vi "Acquisition.vi"(7 "Name(\"\" to use uuid)":string="Acquisition") -> ()   [LabVIEW 2017, in "Acquisition.lvlib"]
uses:
  Acquisition.lvlib
  _support/Hardware Configuration.ctl
  _support/Signal Type.ctl
  bc6f9ce3-7135-4df3-9fce-67397201bd09.vi
  f3e3012a-dc83-45d7-82c5-490bef76f43f.vi
  e2413101-be31-4c43-921b-7e7496268bc5.vi
  07cbb487-6694-43fd-ac53-f2be3466fcff.vi
  fecb174d-6823-407c-a974-ffebb4610b14.vi
  0bf643a1-791c-4b4c-b91f-da80b9c7e2fb.vi
  041ba748-83ae-40d3-86c4-8e2f4b565384.vi
  <userlib>/_NEVSTOP/Communicable State Machine(CSM)/AdvanceAPI/CSM - Revert Arguments-Safe String.vi
  <userlib>/_NEVSTOP/Communicable State Machine(CSM)/_Shared/Trim Single-line Text.vi
  <userlib>/_NEVSTOP/Communicable State Machine(CSM)/AdvanceAPI/CSM - Make String Arguments Safe.vi
  <userlib>/_NEVSTOP/Communicable State Machine(CSM)/AdvanceAPI/CSM - Break Down Multiple States String.vi
  <userlib>/_NEVSTOP/Communicable State Machine(CSM)/AdvanceAPI/CSM - Compact Multiple States.vi
  f3e3012a-dc83-45d7-82c5-490bef76f43f.vi/99de0c97-112a-4c86-9094-c187659127e1.vi
  <userlib>/_NEVSTOP/Communicable State Machine(CSM)/Utility/Build Error Cluster.vi
  0bf643a1-791c-4b4c-b91f-da80b9c7e2fb.vi/99de0c97-112a-4c86-9094-c187659127e1.vi
  <userlib>/_NEVSTOP/Communicable State Machine(CSM)/AdvanceAPI/CSM - Keywords.vi
  <vilib>/Utility/Data Type/Get Type Information.vi
  <userlib>/_NEVSTOP/Communicable State Machine(CSM)/addons/API-String-Arugments-Support/_Support/Data To SingleElementsArray_csm.vi
  <userlib>/_NEVSTOP/Communicable State Machine(CSM)/addons/API-String-Arugments-Support/_Support/Data To API String Arguments.vi
  <userlib>/_NEVSTOP/Communicable State Machine(CSM)/addons/INI-Static-Variable-Support/_Support/Parse Used Session and Name.vi
  <userlib>/_NEVSTOP/Communicable State Machine(CSM)/addons/INI-Static-Variable-Support/_Support/INI-FGV(lvlibp).vi
  <userlib>/_NEVSTOP/Communicable State Machine(CSM)/addons/INI-Static-Variable-Support/_Support/Populate String with INI Variable.vi
  <userlib>/_NEVSTOP/Communicable State Machine(CSM)/addons/API-String-Arugments-Support/_Support/Convert API String Arguments to Data(variant).vi
  <userlib>/_NEVSTOP/Communicable State Machine(CSM)/addons/API-String-Arugments-Support/_Support/SingleElementsArray To Data_csm.vi
  <userlib>/_NEVSTOP/Communicable State Machine(CSM)/addons/API-String-Arugments-Support/_Support/Query Data as API String Arguments(variant).vi
  <userlib>/_NEVSTOP/Communicable State Machine(CSM)/addons/MassData-Parameter/_support/FGV-MassData(lvlibp).vi
  <userlib>/_NEVSTOP/Communicable State Machine(CSM)/_Polymophic/Add State(s) to Queue By BOOL(Element).vi
  <userlib>/_NEVSTOP/Communicable State Machine(CSM)/_Polymophic/CSM - Filter Duplicated Lines.vi
  <userlib>/_NEVSTOP/Communicable State Machine(CSM)/_Polymophic/CSM - Replace Marks in Messages.vi
  <userlib>/_NEVSTOP/Communicable State Machine(CSM)/Communicable State Machine.lvlib
  <userlib>/_NEVSTOP/Communicable State Machine(CSM)/addons/Loop-Support/CSM Loop Support.lvlib
  <userlib>/_NEVSTOP/Communicable State Machine(CSM)/_Shared/CSM Shared.lvlib
panel:
  in  "Signal Type":enum16{"Sine Wave", "Square with Noise"}(ring)
  in  "Cancel Button":bool
  in  "OK Button":bool
  out "Error Occurred":errorcluster
  out "State History":string
  # "Configure The Simulated Waveform Type"
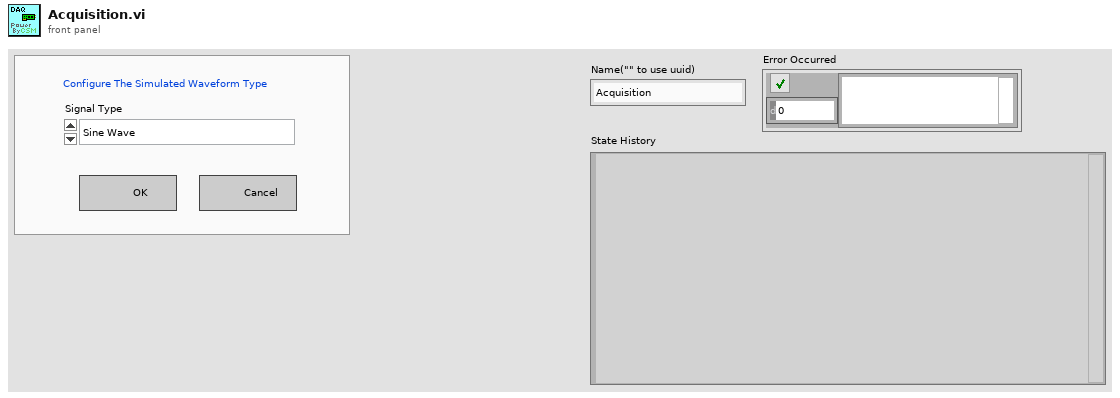
[diagram p1: front panel]
types:
  T1 = enum32{"Invalid", "Default", "Floating", "Floating/Auto-Hide", "Modal"}
  T2 = typedef "Acquisition.lvlib/Hardware Configuration.ctl" = cluster{"Resource":string, "SignalType":T3}
  T3 = typedef "Acquisition.lvlib/Signal Type.ctl" = enum16{"Sine Wave", "Square with Noise"}
  T4 = enum32{"Invalid", "Standard", "Closed", "Hidden", "Minimized", "Maximized"}
  T5 = enum32{"invalid app kind", "Development System", "Run Time System", "Student Edition", "Embedded LabVIEW", "Evaluation", "Custom"}
  T6 = typedef "Communicable State Machine.lvlib/_CSM_Response Source Message.ctl" = cluster{"‘State":string, "’Arguments":string, "’Error":errorcluster}
  T7 = cluster{"Current VI Reference":refnum<vi>, "Close Panel on Exit?":bool}
  T8 = cluster{"Core":cluster{"Current VI Reference":refnum<vi>, "Close Panel on Exit?":bool}, "Configuration":T2, "State":enum16{"Idle", "Acquiring"}, "SamplePeroid(ms)":u32}
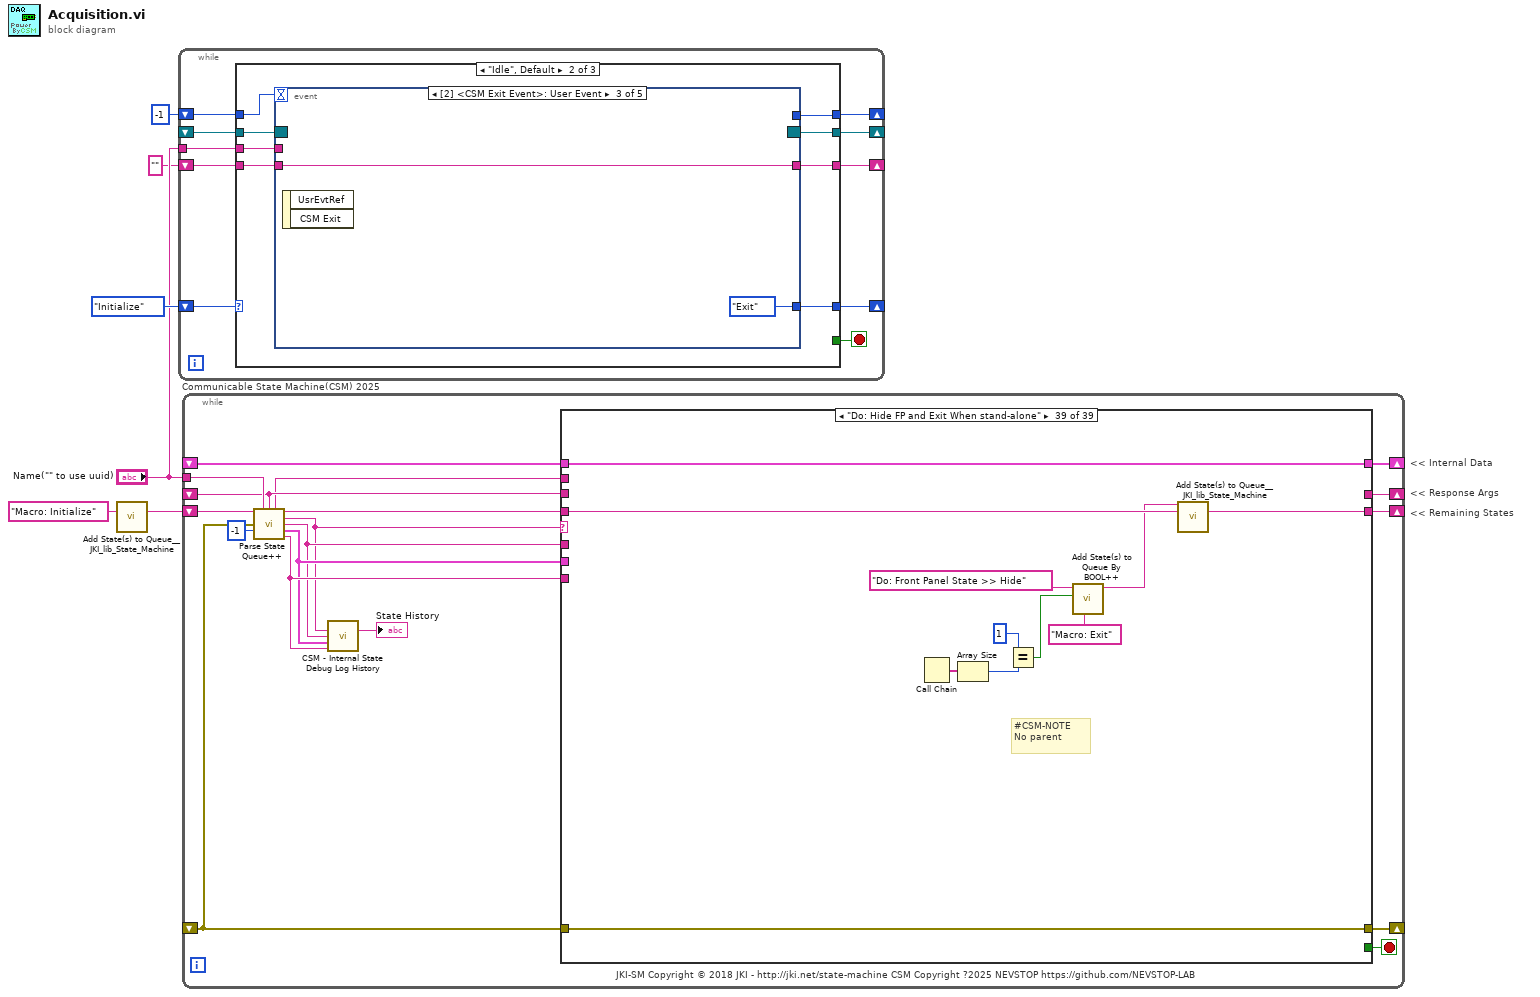
[diagram p0: block diagram]
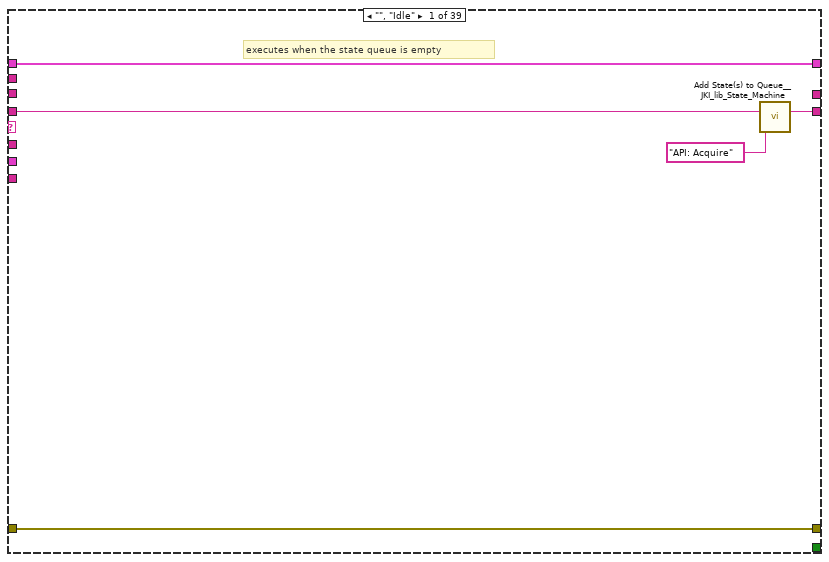
[diagram p2: hidden frame]
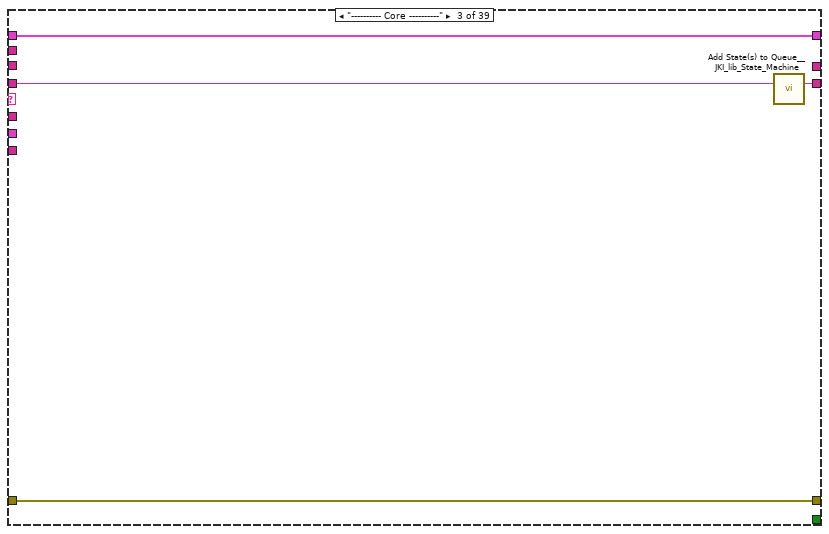
[diagram p4: hidden frame]
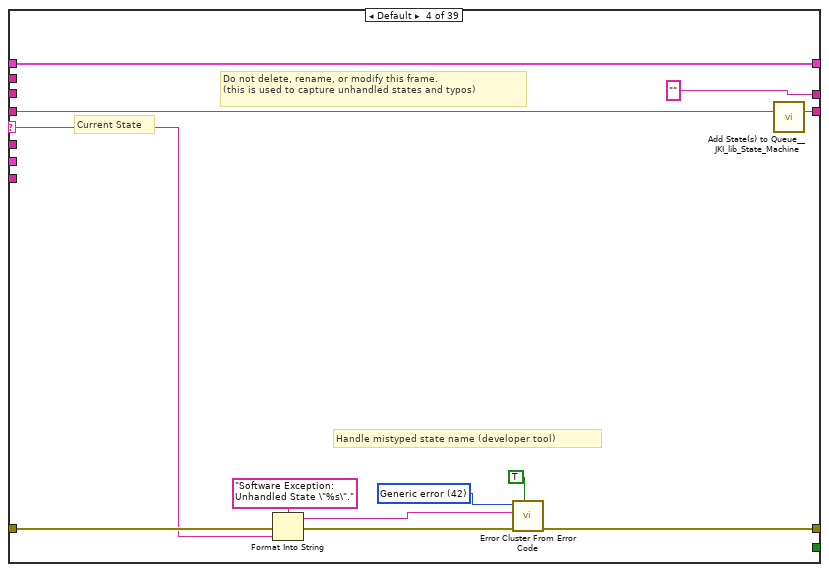
[diagram p5: hidden frame]
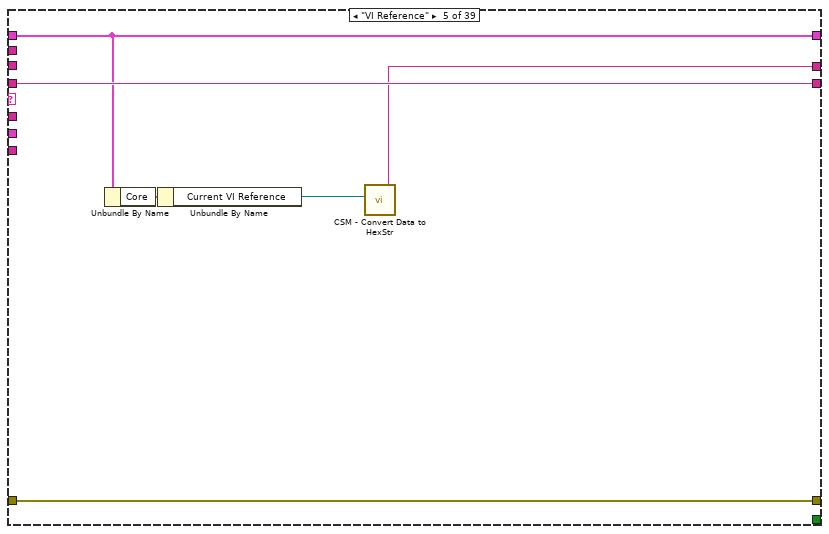
[diagram p6: hidden frame]
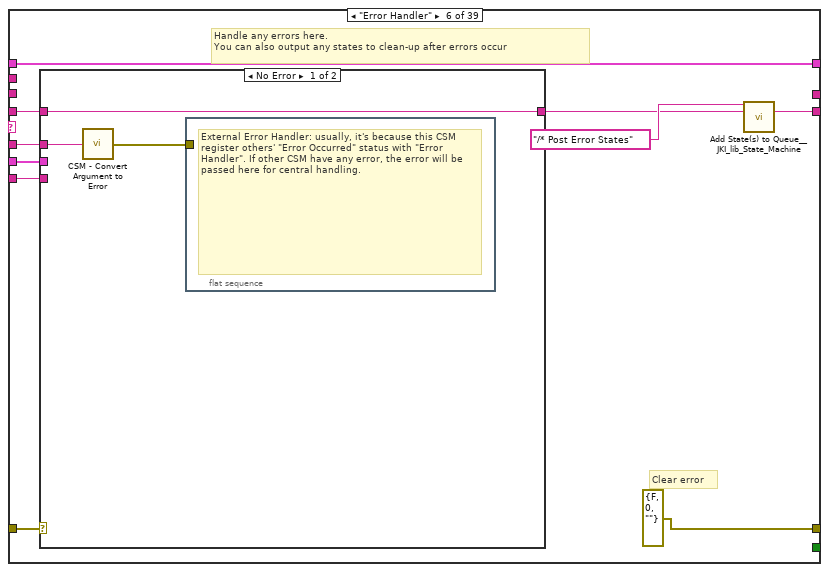
[diagram p7: hidden frame]
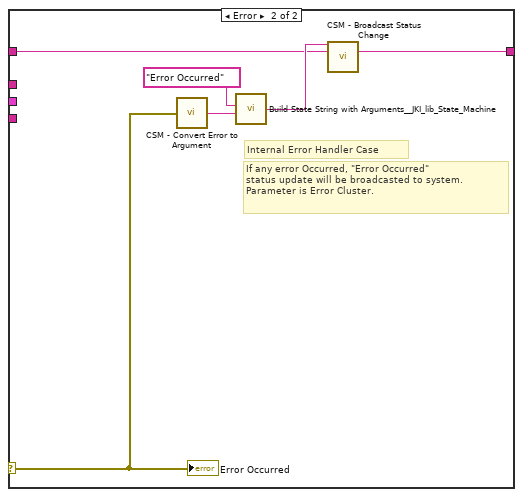
[diagram p8: hidden frame]
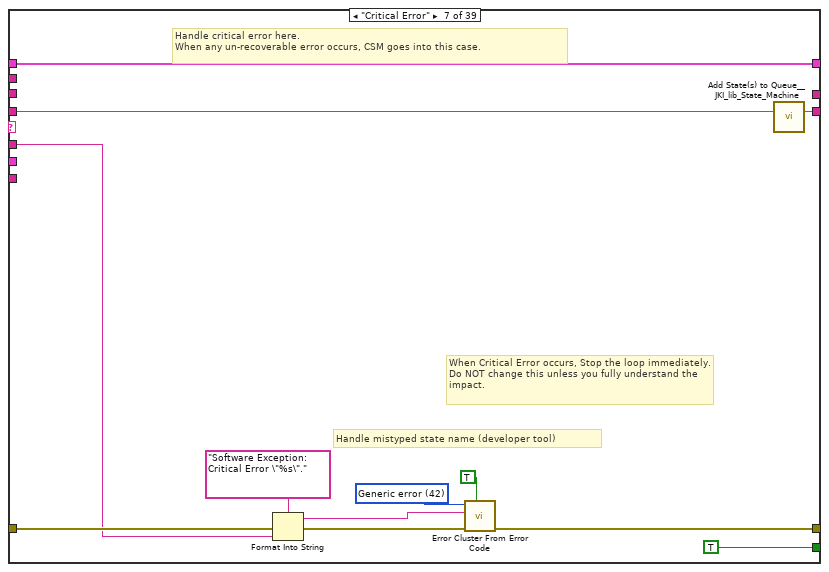
[diagram p9: hidden frame]
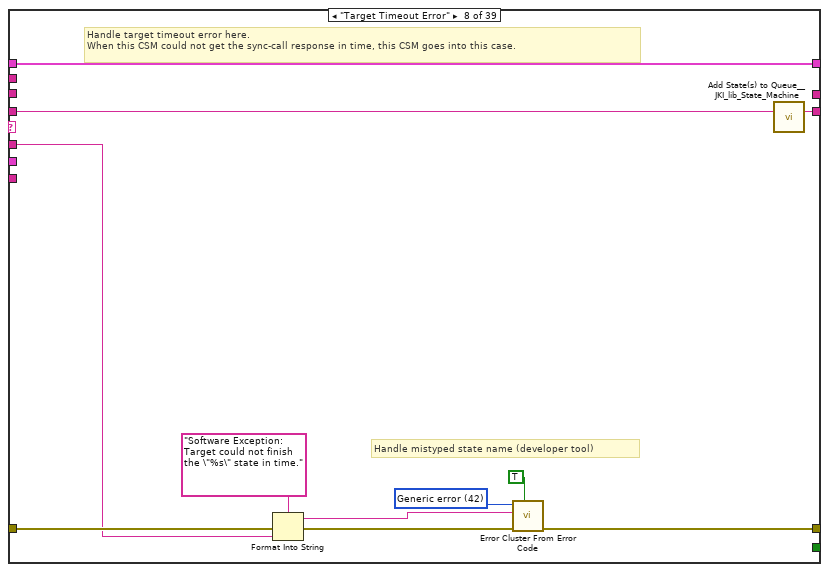
[diagram p10: hidden frame]
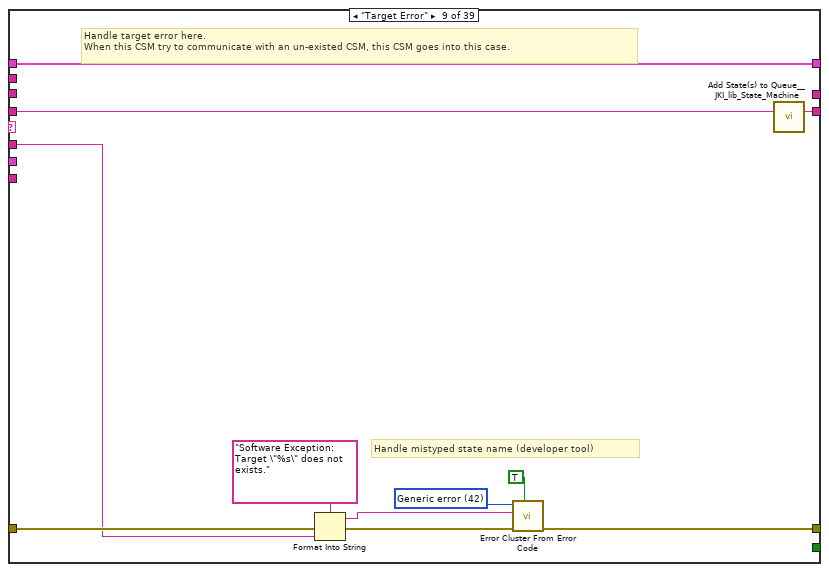
[diagram p11: hidden frame]
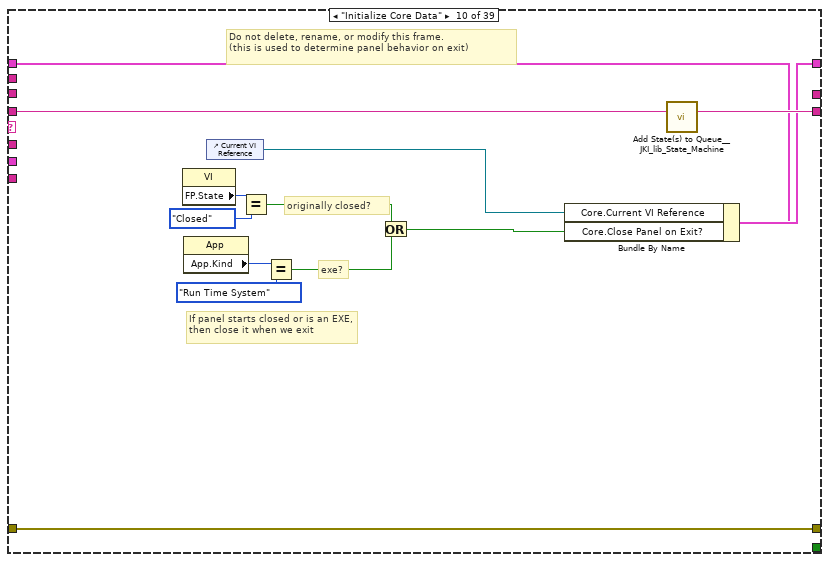
[diagram p12: hidden frame]
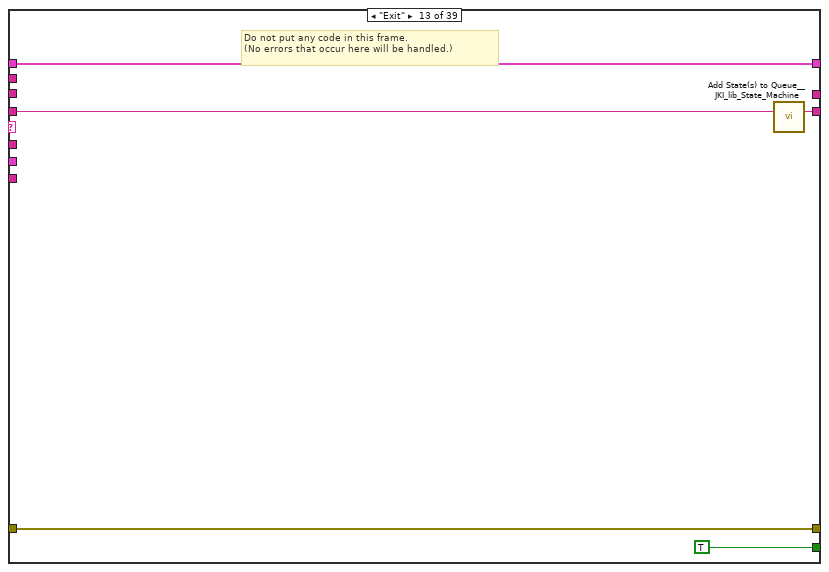
[diagram p15: hidden frame]
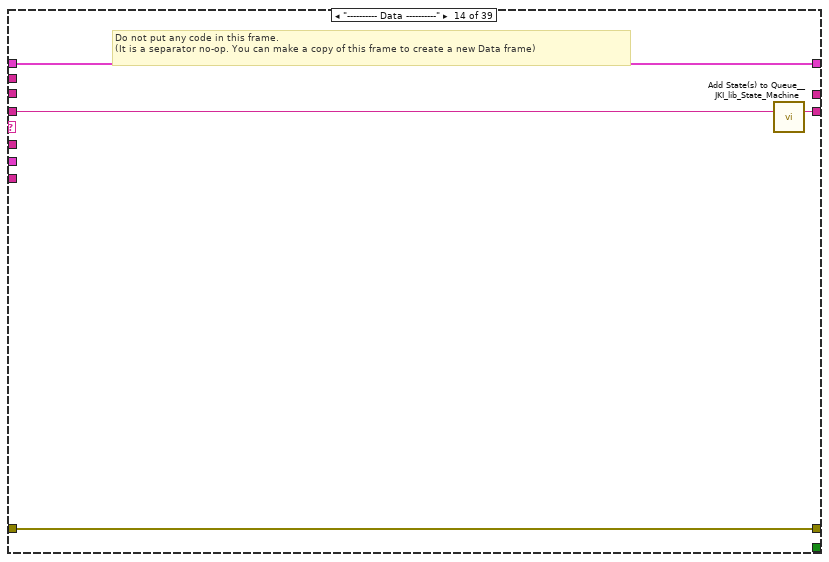
[diagram p16: hidden frame]
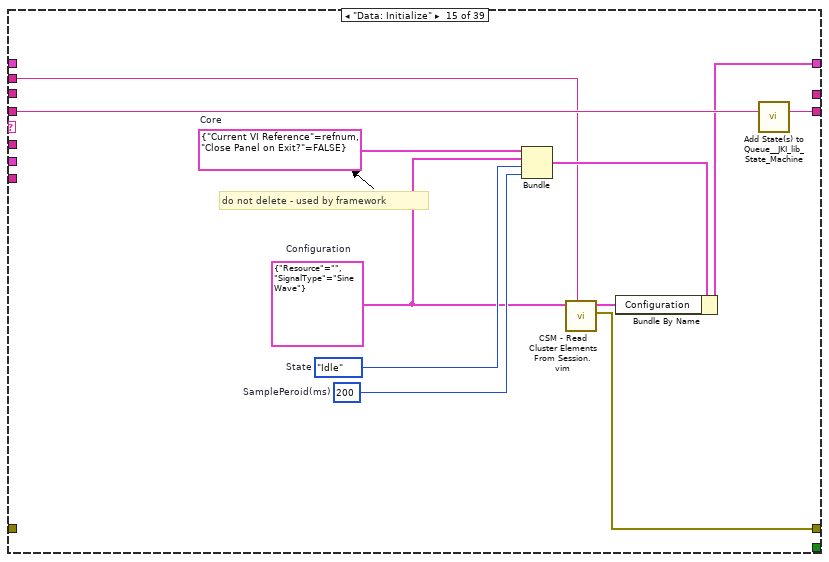
[diagram p17: hidden frame]
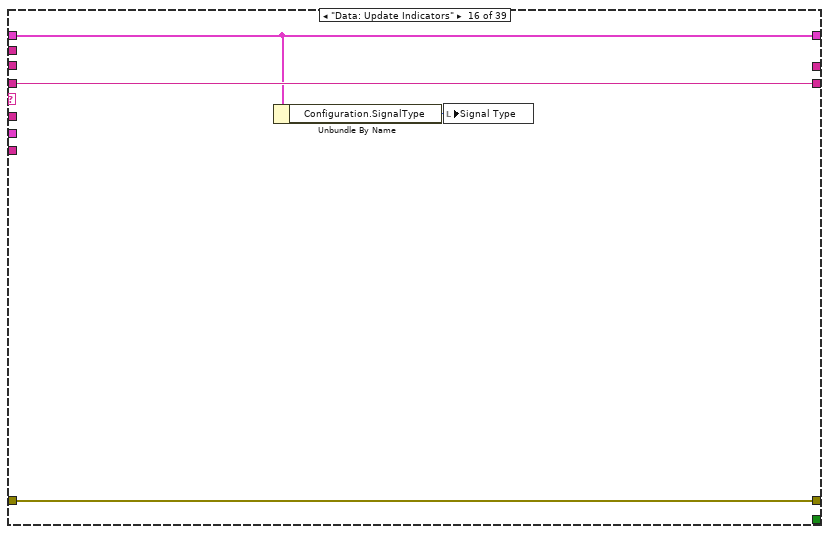
[diagram p18: hidden frame]
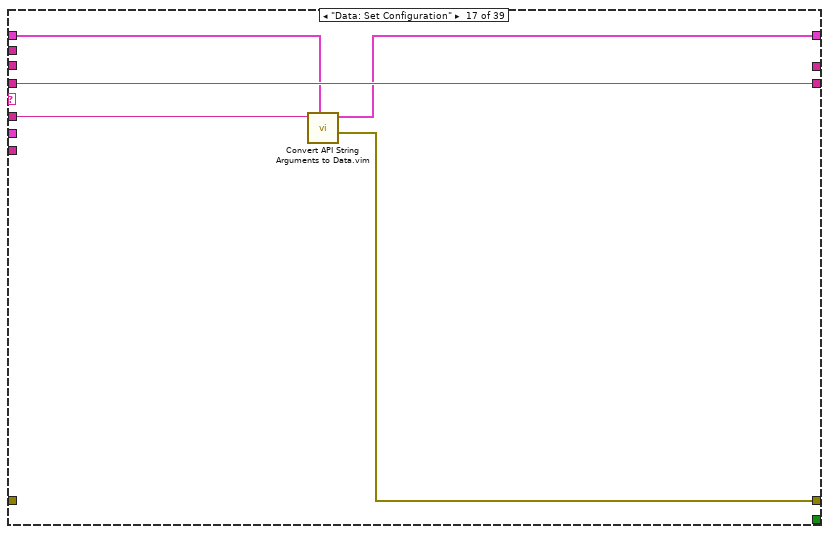
[diagram p19: hidden frame]
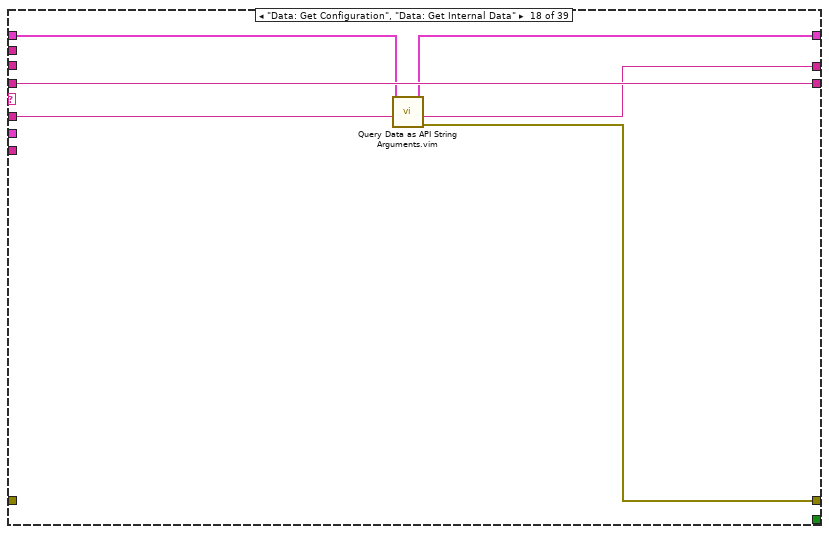
[diagram p20: hidden frame]
diagram:
  # "<< Internal Data"
  # "<< Response Args"
  # "<< Remaining States"
  n1 = call <vilib>:"Add State(s) to Queue__JKI_lib_State_Machine.vi"("State(s) in (\"\")"="Macro: Initialize") -> ("States Out"=w5:string)  [unwired: 14 in]
  n2 = while {
    shift-right: [w12] -> _
    shift-left: enum16{"Idle", "Initialize", "Exit"}."Initialize" -> [w16]
    tunnel: "Name(\"\" to use uuid)" -> [w15]
    shift-right: [w14] -> _
    shift-left: _ -> [w13]
    shift-right: [w9] -> _
    shift-left: "" -> [w10]
    shift-right: [w7] -> _
    shift-left: -1 -> [w8]
    stop <- w11 stop-if-true
    n3 = case shown="\"Idle\", Default" w16 {
      tunnel: w15 -> [w25 w29 _]
      tunnel: [w22 w34 _] -> w14
      tunnel: w13 -> [_ w33 w62]
      tunnel: [enum16{"Idle", "Initialize", "Exit"}."Idle" w32 _] -> w12
      tunnel: [_ _ TRUE] -> w11
      tunnel: w10 -> [w19 w31 w59]
      tunnel: [w19 w30 w59] -> w9
      tunnel: w8 -> [w18 w27 w58]
      tunnel: [w18 w28 w58] -> w7
      frame "Initialize" {
        n4 = call <userlib>:"CSM - Wait for Module to Be Alive.vi"("CSM Name"=w25) -> ("CSM Name (Dup)"=w20:string, "error out"=w26:errorcluster)  [unwired: 12 in, 1 out]
        n5 = call <userlib>:"CSM - Module Exit Event.vi"("Error In"=w26, "Name (\"\" to Use UUID) In"=w20) -> ("error out"=w24:errorcluster, "CSM Exit Event"=w23:refnum<user-event>)  [unwired: 7 in, 1 out]
        n6 = register-events(error in=w24, w23) -> (reference out=w22:refnum<event-registration>)  [unwired: 1 in, 1 out]
        n7 = property class="VI"("FP.Behavior"=T1."Default" ("Front Panel Window:Behavior")) -> ()  [unwired: 2 in, 2 out]
      }
      frame "Idle", Default {
        n8 = event shown="[2] <CSM Exit Event>: User Event" {
          selector: w33 -> [_ _ _ _ _]
          dyn-events: [_ _ _ _ _] -> w34
          timeout: w27 -> [_ _ _ _ _]
          tunnel: [_ _ enum16{"Idle", "Initialize", "Exit"}."Exit" _ _] -> w32
          tunnel: w31 -> [w38 w42 w44 w53 w56]
          tunnel: [w39 w41 w44 w52 w55] -> w30
          tunnel: w29 -> [w36 _ _ _ _]
          tunnel: [-1 _ _ _ _] -> w28
          event Timeout {
            n9 = event-data() -> ()  [unwired: 1 in, 3 out]
            n10 = call-poly <userlib>:"CSM - Filter JKISM String Queue.vi"("States In"=w38) -> ("States Out"=w35:string)  [unwired: 14 in]
            n11 = call <userlib>:"CSM - Forward UI Operations to CSM.vi"("Name (\"\" to Use UUID)"=w36, "State(s) In (\"\")"=w35) -> ("States Out"=w39:string)  [unwired: 8 in, 1 out]
          }
          event Panel Close? {
            n12 = event-data() -> ()  [unwired: 1 in, 2 out]
            n13 = call <vilib>:"Add State(s) to Queue__JKI_lib_State_Machine.vi"("State(s) in Front (\"\")"="Do: Hide FP and Exit When stand-alone" ("State(s) in Front (\"\")"), "State(s) in (\"\")"=w42) -> ("States Out"=w41:string)  [unwired: 13 in]
            n14 = event-data("Discard?"=TRUE) -> ()  [unwired: 1 in, 1 out]
          }
          event User Event {
            n15 = event-data() -> ()  [unwired: 1 in, 2 out]
          }
          event "OK Button": Value Change {
            n16 = event-data() -> ()  [unwired: 1 in, 1 out]
            n17 = Bundle By Name(cluster=T2 {"Resource"="", "SignalType"=enum."Sine Wave"} ("Hardware Config"), "SignalType"="Signal Type") -> (w48:T2)
            n18 = call "Convert Data To API String Arguments.vim"("Data"=w48) -> ("API String"=w47:string)  [unwired: 7 in, 1 out]
            n19 = call-poly <userlib>:"Build Message with Arguments++.vi"("States With Replace Token"="API: Update Settings >> <param>\nData: Update Indicators\nDo: Hide FP and Exit When stand-alone" ("State"), "<param>"=w47) -> ("States"=w46:string)  [unwired: 13 in]
            n20 = call <vilib>:"Add State(s) to Queue__JKI_lib_State_Machine.vi"("State(s) in (\"\")"=w53, "State(s) at Back (\"\")"=w46) -> ("States Out"=w52:string)  [unwired: 13 in]
          }
          event "Cancel Button": Value Change {
            n21 = event-data() -> ()  [unwired: 1 in, 1 out]
            n22 = call <vilib>:"Add State(s) to Queue__JKI_lib_State_Machine.vi"("State(s) in Front (\"\")"="Do: Hide FP and Exit When stand-alone" ("State(s) in Front (\"\")"), "State(s) in (\"\")"=w56) -> ("States Out"=w55:string)  [unwired: 13 in]
          }
        }
      }
      frame "Exit" {
        n23 = Unregister For Events(event registration refnum=w62) -> (error out=w61:errorcluster)  [unwired: 1 in]
        n24 = call <vilib>:"Clear Errors.vi"("error in (no error)"=w61) -> ()  [unwired: 5 in, 2 out]
        n25 = property class="VI"("FP.Behavior"=T1."Default" ("Front Panel Window:Behavior")) -> ()  [unwired: 2 in, 2 out]
      }
    }
  }
  n26 = while "Communicable State Machine(CSM) 2025" {
    shift-right: [w75] -> _
    shift-left: _ -> [w65]
    shift-right: [w78] -> _
    shift-left: _ -> [w74]
    shift-right: [w77] -> _
    shift-left: w5 -> [w79]
    tunnel: "Name(\"\" to use uuid)" -> [w72]
    shift-right: [w73] -> _
    shift-left: _ -> [w67]
    stop <- w76 stop-if-true
    # "JKI-SM Copyright © 2018 JKI - http://jki.net/state-machine CSM Copyright ?2025 NEVSTOP https://github.com/NEVSTOP-LAB"
    n27 = call <userlib>:"Parse State Queue++.vi"("State Queue"=w79, "Name (\"\" to Use UUID)"=w72, "Response Arguments"=w67, "Previous Error"=w74, "Dequeue (1 ms)"=-1 ("Dequeue Timeout(1ms)")) -> ("Name Used"=w66:string, "Remaining States"=w80:string, "Current State"=w68:string, "Arguments"=w69:string, "Additional Information"=w70:T6, "Source CSM"=w71:string)  [unwired: 5 in]
    n28 = call <userlib>:"CSM - Internal State Debug Log History.vi"("State"=w68, "Arguments (\"\")"=w69, ">> Response Source Message >>"=w70, "Source (\"\")"=w71) -> ("Debug Log"=→"State History":string)  [unwired: 11 in]
    n29 = case shown="\"Do: Hide FP and Exit When stand-alone\"" w68 {
      selector: w68 -> [_ _ _ w94 _ _ _ _ _ _ _ _ _ _ _ _ _ _ _ _ _ _ _ _ _ _ _ _ _ _ _ _ _ _ w334 _ _ _ _]
      tunnel: w80 -> [w82 w87 w92 w98 w109 w114 w135 w147 w158 w176 w178 w181 w187 w191 w202 w205 w211 w217 w223 w227 w232 w237 w239 w243 w256 w269 w280 w287 w293 w298 w303 w326 w328 w331 w338 w341 w345 w352 w419]
      tunnel: w69 -> [_ _ _ _ _ w113 w131 w143 w154 _ _ _ _ _ _ _ w209 w214 _ _ _ _ _ _ _ w265 _ _ _ _ _ _ _ _ w333 _ _ w349 _]
      tunnel: w65 -> [w84 w86 w89 w96 w108 w119 w133 w145 w156 w169 w177 w180 w185 w188 _ w203 w210 w216 w218 w224 w229 w234 w238 w246 w252 w267 w279 w285 w290 w297 w305 w323 w327 w330 w336 w342 w344 w351 w428]
      tunnel: [w85 w88 w90 w100 w110 errorcluster {"status"=FALSE, "code"=0, "source"=""} ("error out") w137 w142 w153 w173 w179 w182 w184 w189 w192 w206 w207 w212 w219 w225 w230 w235 w240 w244 w254 w261 w281 w282 w288 w299 w307 w324 w329 w332 w339 w343 w346 w348 w427] -> w78
      tunnel: w74 -> [w85 w88 w90 w99 w110 w117 w136 w148 w159 w173 w179 w182 w184 w189 _ w206 _ _ w220 w225 w230 w235 w240 w244 w254 _ w281 _ _ w299 w308 _ w329 w332 w339 w343 w346 w350 w427]
      tunnel: [w83 w87 w91 w97 w109 w115 w134 w146 w157 w175 w178 w181 w186 w190 w201 w205 w211 w217 w222 w226 w231 w236 w239 w242 w255 w269 w280 w287 w293 w298 w304 w326 w328 w331 w337 w340 w345 w352 w420] -> w77
      tunnel: [_ _ _ _ _ _ TRUE _ _ _ _ _ TRUE _ _ _ _ _ _ _ _ _ _ _ _ _ _ _ _ _ _ _ _ _ _ _ _ _ _] -> w76
      tunnel: [w84 w86 w89 w96 w108 w119 w133 w145 w156 w174 w177 w180 w185 w188 w194 w203 w208 w215 w218 w224 w229 w234 w238 w245 w252 w268 w279 w283 w289 w296 w306 w322 w327 w330 w336 w342 w344 w351 w428] -> w75
      tunnel: w71 -> [_ _ _ _ _ w112 _ _ _ _ _ _ _ _ _ _ _ _ _ _ _ _ _ _ _ _ _ _ _ _ _ _ _ _ _ _ _ _ _]
      tunnel: w70 -> [_ _ _ _ _ w111 _ _ _ _ _ _ _ _ _ _ _ _ _ _ _ _ _ _ _ _ _ _ _ _ _ _ _ _ _ _ _ _ _]
      tunnel: [_ _ _ "" w105 _ _ _ _ _ _ _ _ _ _ _ _ w213 _ _ _ _ _ _ _ _ _ _ _ _ w301 _ _ _ _ _ _ _ _] -> w73
      tunnel: w66 -> [_ _ _ _ _ _ _ _ _ _ _ _ _ _ w196 _ _ _ _ _ _ _ _ _ _ w260 _ _ _ _ _ _ _ _ _ _ _ _ _]
      tunnel: w67 -> [_ _ _ _ _ _ _ _ _ _ _ _ _ _ _ _ _ _ _ _ _ _ _ _ _ _ _ _ _ _ _ _ _ _ _ _ _ _ _]
      frame "", "Idle" {
        # "executes when the state queue is empty"
        n30 = call <vilib>:"Add State(s) to Queue__JKI_lib_State_Machine.vi"("State(s) in (\"\")"=w82, "State(s) at Back (\"\")"="API: Acquire" ("State(s) in Front (\"\")")) -> ("States Out"=w83:string)  [unwired: 13 in]
      }
      frame "CSM Documentation" {
        # "CSM Documentation"
        # "State Syntax:\nStateCategory: State >> Argument -@ CSMName\nStateCategory: State >> Argument -> CSMName\n\nLine Terminator: Line feed"
        # "Commenting:\nTo add a comment use \"//\" or \"#\" and all text to the right will be ignored\nCommenting Example:\nUI: Initialize // This initializes the UI\n// Another comment line"
        # "Example:\nUI: Help >> About -@Main\nUI: Help >> About ->Main\n\nWhere \"UI\" is the state category\nWhere \"Help\" is the state\nWhere \"About\" is the argument\nWhere \"Main\" is the Name of CSM,which actually run the \"UI: Help >> About\"\n\n    \"-@\" stands for sync state. Current CSM will wait until the state is finished. \n            - if \"Main\" named CSM does not exist, \"Target Error\" will occur.\n            - if \"Main\" named CSM is in another sync remote state, \"Target Busy Error\" will occur.\n            - if \"Main\" named CSM could not finish the state in time, \"Target Timeout Error\" will occur.\n            - if everything is right. \"Response\" will occur with Argument back from \"Main\" named CSM. \n\n    \"->\" stands for async state. Current CSM will post the state and continue to next state in next iteration.\n            - if \"Main\" named CSM does not exist, \"Target Error\" will occur.\n            - if everything is right. \"Async Message Posted\" will occur.\n            - After State is finished. Caller will receive a \"Async Response\" state from callee.\n\nWhen duplicated name is used for multiple CSM module or some framework problem happens, \"Critical Error\" will occur."
      }
      frame "---------- Core ----------" {
        n31 = call <vilib>:"Add State(s) to Queue__JKI_lib_State_Machine.vi"("State(s) in (\"\")"=w92) -> ("States Out"=w91:string)  [unwired: 14 in]
      }
      frame Default {
        w103 = 42 items=["No error", "Argument error", "Memory is full", "Out of zone", "End of file", "File already open", "Generic file I/O error", "File not found", "File permission error", "Disk is full", "Duplicate path", "Too many files open", "System feature not enabled", "Resource file not found", "Cannot add resource", "Resource not found", "Image not found", "Image memory error", "Pen does not exist", "Config type invalid", "Config token not found", "Config parse error", "Config memory error", "Bad external code format", "Bad external code offset", "External code not present", "Null window", "Destroy window error", "Null menu", "Print aborted", "Bad print record", "Print driver error", "Windows error during printing", "Memory error during printing", "Print dialog error", "Generic print error", "Invalid device refnum", "Device not found", "Device parameter error", "Device unit error", "Cannot open device", "Device call aborted", "Generic error", "Cancelled by user", "Object ID too low", "Object ID too high", "Object not in heap", "Unknown heap", "Unknown object (invalid DefProc)", "Unknown object (DefProc not in table)", "Message out of range", "Invalid (null) method", "Unknown message", "Manager call not supported", "Bad address", "Network operation in progress", "Network operation timed out", "Connection is busy", "Network attribute not supported", "Network error", "Address in use", "System out of memory", "Connection aborted", "Connection refused", "Not connected", "Already connected", "Connection closed", "Initialization error (interapplication manager)", "Bad occurrence", "Wait on unbound occurrence handler", "Occurrence queue overflow", "Datalog type conflict", "Unused", "Unrecognized type (interapplication manager)", "Memory corrupt", "Failed to make temporary DLL", "Old CIN version", "Drag socket not found", "Failed to load drop-object", "Failed to register OLE object", "Failed to release OLE object", "Format specifier type mismatch", "Unknown format specifier", "Too few format specifiers", "Too many format specifiers", "Scan failed", "Newer CIN version", "Error converting to variant", "Runtime menu error", "Password tampered", "Variant attribute not found", "Incompatible variant data type", "Event data is not available", "Event Store is not present", "Occurrence is not found", "Event Queue is not created", "Event info is not available", "Refnum passed is NULL", "Error retrieving Class GUID", "Error retrieving CoClass GUID", "Error retrieving TypeLib GUID.", "Bad built application magic bytes.", "Specific driver is different from the specific driver associated with the Logical Name.", "There is no session opened to the class driver.", "Max Error", "MAX - Error with config objects", "MAX - Error loading configuration", "MAX - Group not supported"]
        # "Current State"
        # "Do not delete, rename, or modify this frame.\n(this is used to capture unhandled states and typos)"
        # "Handle mistyped state name (developer tool)"
        n32 = Format Into String(format string="Software Exception: Unhandled State \"%s\"." ("message"), error in=w99, w94) -> (resulting string=w102:string, error out=w101:errorcluster)  [unwired: 1 in]
        n33 = call <vilib>:"Error Cluster From Error Code.vi"("show call chain? (False)"=TRUE, "error in (no error)"=w101, "error message (\"\")"=w102, "error code (0)"=w103) -> ("error out"=w100:errorcluster)  [unwired: 5 in]
        n34 = call <vilib>:"Add State(s) to Queue__JKI_lib_State_Machine.vi"("State(s) in (\"\")"=w98) -> ("States Out"=w97:string)  [unwired: 14 in]
      }
      frame "VI Reference" {
        n35 = Unbundle By Name(w108) -> ("Core"=w107:T7)
        n36 = Unbundle By Name(w107) -> ("Current VI Reference"=w106:refnum<vi>)
        n37 = call <userlib>:"CSM - Convert Data to HexStr.vi"("Variant"=w106) -> ("HEX String (0-9,A-F)"=w105:string)  [unwired: 8 in]
      }
      frame "Error Handler" {
        # "Handle any errors here.\nYou can also output any states to clean-up after errors occur"
        # "Clear error"
        n38 = case shown="No Error" w117 {
          selector: w117 -> [_ w124]
          tunnel: [w123 w126] -> w116
          tunnel: w114 -> [w123 w125]
          tunnel: w113 -> [w122 _]
          tunnel: w112 -> [_ _]
          tunnel: w111 -> [_ _]
          frame No Error {
            n39 = call <userlib>:"CSM - Convert Argument to Error.vi"("Argument"=w122) -> ("Error"=w121:errorcluster)  [unwired: 4 in]
            n40 = flat-sequence {
              tunnel: w121 -> [_]
              frame #0 {
                # "External Error Handler: usually, it's because this CSM register others' \"Error Occurred\" status with \"Error Handler\". If other CSM have any error, the error will be passed here for central handling."
              }
            }
          }
          frame Error {
            # "Internal Error Handler Case"
            # "If any error Occurred, \"Error Occurred\" \nstatus update will be broadcasted to system.\nParameter is Error Cluster."
            n41 = call <userlib>:"CSM - Convert Error to Argument.vi"("Error"=w124) -> ("Argument"=w128:string)  [unwired: 4 in]
            n42 = call <vilib>:"Build State String with Arguments__JKI_lib_State_Machine.vi"("Arguments (\"\")"=w128, "State"="Error Occurred" ("Status with Arguments")) -> ("State with Arguments"=w127:string)  [unwired: 4 in]
            n43 = call <userlib>:"CSM - Broadcast Status Change.vi"("Status With Arguments"=w127, "State Queue"=w125) -> ("Remaining States"=w126:string)  [unwired: 13 in]
            "Error Occurred" <- w124
          }
        }
        n44 = call <vilib>:"Add State(s) to Queue__JKI_lib_State_Machine.vi"("State(s) in Front (\"\")"="/* Post Error States", "State(s) in (\"\")"=w116) -> ("States Out"=w115:string)  [unwired: 13 in]
      }
      frame "Critical Error" {
        w140 = 42 items=["No error", "Argument error", "Memory is full", "Out of zone", "End of file", "File already open", "Generic file I/O error", "File not found", "File permission error", "Disk is full", "Duplicate path", "Too many files open", "System feature not enabled", "Resource file not found", "Cannot add resource", "Resource not found", "Image not found", "Image memory error", "Pen does not exist", "Config type invalid", "Config token not found", "Config parse error", "Config memory error", "Bad external code format", "Bad external code offset", "External code not present", "Null window", "Destroy window error", "Null menu", "Print aborted", "Bad print record", "Print driver error", "Windows error during printing", "Memory error during printing", "Print dialog error", "Generic print error", "Invalid device refnum", "Device not found", "Device parameter error", "Device unit error", "Cannot open device", "Device call aborted", "Generic error", "Cancelled by user", "Object ID too low", "Object ID too high", "Object not in heap", "Unknown heap", "Unknown object (invalid DefProc)", "Unknown object (DefProc not in table)", "Message out of range", "Invalid (null) method", "Unknown message", "Manager call not supported", "Bad address", "Network operation in progress", "Network operation timed out", "Connection is busy", "Network attribute not supported", "Network error", "Address in use", "System out of memory", "Connection aborted", "Connection refused", "Not connected", "Already connected", "Connection closed", "Initialization error (interapplication manager)", "Bad occurrence", "Wait on unbound occurrence handler", "Occurrence queue overflow", "Datalog type conflict", "Unused", "Unrecognized type (interapplication manager)", "Memory corrupt", "Failed to make temporary DLL", "Old CIN version", "Drag socket not found", "Failed to load drop-object", "Failed to register OLE object", "Failed to release OLE object", "Format specifier type mismatch", "Unknown format specifier", "Too few format specifiers", "Too many format specifiers", "Scan failed", "Newer CIN version", "Error converting to variant", "Runtime menu error", "Password tampered", "Variant attribute not found", "Incompatible variant data type", "Event data is not available", "Event Store is not present", "Occurrence is not found", "Event Queue is not created", "Event info is not available", "Refnum passed is NULL", "Error retrieving Class GUID", "Error retrieving CoClass GUID", "Error retrieving TypeLib GUID.", "Bad built application magic bytes.", "Specific driver is different from the specific driver associated with the Logical Name.", "There is no session opened to the class driver.", "Max Error", "MAX - Error with config objects", "MAX - Error loading configuration", "MAX - Group not supported"]
        # "Handle critical error here.\nWhen any un-recoverable error occurs, CSM goes into this case."
        # "When Critical Error occurs, Stop the loop immediately. Do NOT change this unless you fully understand the impact."
        # "Handle mistyped state name (developer tool)"
        n45 = Format Into String(format string="Software Exception: Critical Error \"%s\"." ("message"), error in=w136, w131) -> (resulting string=w139:string, error out=w138:errorcluster)  [unwired: 1 in]
        n46 = call <vilib>:"Error Cluster From Error Code.vi"("show call chain? (False)"=TRUE, "error in (no error)"=w138, "error message (\"\")"=w139, "error code (0)"=w140) -> ("error out"=w137:errorcluster)  [unwired: 5 in]
        n47 = call <vilib>:"Add State(s) to Queue__JKI_lib_State_Machine.vi"("State(s) in (\"\")"=w135) -> ("States Out"=w134:string)  [unwired: 14 in]
      }
      frame "Target Timeout Error" {
        w151 = 42 items=["No error", "Argument error", "Memory is full", "Out of zone", "End of file", "File already open", "Generic file I/O error", "File not found", "File permission error", "Disk is full", "Duplicate path", "Too many files open", "System feature not enabled", "Resource file not found", "Cannot add resource", "Resource not found", "Image not found", "Image memory error", "Pen does not exist", "Config type invalid", "Config token not found", "Config parse error", "Config memory error", "Bad external code format", "Bad external code offset", "External code not present", "Null window", "Destroy window error", "Null menu", "Print aborted", "Bad print record", "Print driver error", "Windows error during printing", "Memory error during printing", "Print dialog error", "Generic print error", "Invalid device refnum", "Device not found", "Device parameter error", "Device unit error", "Cannot open device", "Device call aborted", "Generic error", "Cancelled by user", "Object ID too low", "Object ID too high", "Object not in heap", "Unknown heap", "Unknown object (invalid DefProc)", "Unknown object (DefProc not in table)", "Message out of range", "Invalid (null) method", "Unknown message", "Manager call not supported", "Bad address", "Network operation in progress", "Network operation timed out", "Connection is busy", "Network attribute not supported", "Network error", "Address in use", "System out of memory", "Connection aborted", "Connection refused", "Not connected", "Already connected", "Connection closed", "Initialization error (interapplication manager)", "Bad occurrence", "Wait on unbound occurrence handler", "Occurrence queue overflow", "Datalog type conflict", "Unused", "Unrecognized type (interapplication manager)", "Memory corrupt", "Failed to make temporary DLL", "Old CIN version", "Drag socket not found", "Failed to load drop-object", "Failed to register OLE object", "Failed to release OLE object", "Format specifier type mismatch", "Unknown format specifier", "Too few format specifiers", "Too many format specifiers", "Scan failed", "Newer CIN version", "Error converting to variant", "Runtime menu error", "Password tampered", "Variant attribute not found", "Incompatible variant data type", "Event data is not available", "Event Store is not present", "Occurrence is not found", "Event Queue is not created", "Event info is not available", "Refnum passed is NULL", "Error retrieving Class GUID", "Error retrieving CoClass GUID", "Error retrieving TypeLib GUID.", "Bad built application magic bytes.", "Specific driver is different from the specific driver associated with the Logical Name.", "There is no session opened to the class driver.", "Max Error", "MAX - Error with config objects", "MAX - Error loading configuration", "MAX - Group not supported"]
        # "Handle target timeout error here.\nWhen this CSM could not get the sync-call response in time, this CSM goes into this case."
        # "Handle mistyped state name (developer tool)"
        n48 = Format Into String(format string="Software Exception: Target could not finish the \"%s\" state in time." ("message"), error in=w148, w143) -> (resulting string=w150:string, error out=w149:errorcluster)  [unwired: 1 in]
        n49 = call <vilib>:"Error Cluster From Error Code.vi"("show call chain? (False)"=TRUE, "error in (no error)"=w149, "error message (\"\")"=w150, "error code (0)"=w151) -> ("error out"=w142:errorcluster)  [unwired: 5 in]
        n50 = call <vilib>:"Add State(s) to Queue__JKI_lib_State_Machine.vi"("State(s) in (\"\")"=w147) -> ("States Out"=w146:string)  [unwired: 14 in]
      }
      frame "Target Error" {
        w162 = 42 items=["No error", "Argument error", "Memory is full", "Out of zone", "End of file", "File already open", "Generic file I/O error", "File not found", "File permission error", "Disk is full", "Duplicate path", "Too many files open", "System feature not enabled", "Resource file not found", "Cannot add resource", "Resource not found", "Image not found", "Image memory error", "Pen does not exist", "Config type invalid", "Config token not found", "Config parse error", "Config memory error", "Bad external code format", "Bad external code offset", "External code not present", "Null window", "Destroy window error", "Null menu", "Print aborted", "Bad print record", "Print driver error", "Windows error during printing", "Memory error during printing", "Print dialog error", "Generic print error", "Invalid device refnum", "Device not found", "Device parameter error", "Device unit error", "Cannot open device", "Device call aborted", "Generic error", "Cancelled by user", "Object ID too low", "Object ID too high", "Object not in heap", "Unknown heap", "Unknown object (invalid DefProc)", "Unknown object (DefProc not in table)", "Message out of range", "Invalid (null) method", "Unknown message", "Manager call not supported", "Bad address", "Network operation in progress", "Network operation timed out", "Connection is busy", "Network attribute not supported", "Network error", "Address in use", "System out of memory", "Connection aborted", "Connection refused", "Not connected", "Already connected", "Connection closed", "Initialization error (interapplication manager)", "Bad occurrence", "Wait on unbound occurrence handler", "Occurrence queue overflow", "Datalog type conflict", "Unused", "Unrecognized type (interapplication manager)", "Memory corrupt", "Failed to make temporary DLL", "Old CIN version", "Drag socket not found", "Failed to load drop-object", "Failed to register OLE object", "Failed to release OLE object", "Format specifier type mismatch", "Unknown format specifier", "Too few format specifiers", "Too many format specifiers", "Scan failed", "Newer CIN version", "Error converting to variant", "Runtime menu error", "Password tampered", "Variant attribute not found", "Incompatible variant data type", "Event data is not available", "Event Store is not present", "Occurrence is not found", "Event Queue is not created", "Event info is not available", "Refnum passed is NULL", "Error retrieving Class GUID", "Error retrieving CoClass GUID", "Error retrieving TypeLib GUID.", "Bad built application magic bytes.", "Specific driver is different from the specific driver associated with the Logical Name.", "There is no session opened to the class driver.", "Max Error", "MAX - Error with config objects", "MAX - Error loading configuration", "MAX - Group not supported"]
        # "Handle target error here.\nWhen this CSM try to communicate with an un-existed CSM, this CSM goes into this case."
        # "Handle mistyped state name (developer tool)"
        n51 = Format Into String(format string="Software Exception: Target \"%s\" does not exists." ("message"), error in=w159, w154) -> (resulting string=w161:string, error out=w160:errorcluster)  [unwired: 1 in]
        n52 = call <vilib>:"Error Cluster From Error Code.vi"("show call chain? (False)"=TRUE, "error in (no error)"=w160, "error message (\"\")"=w161, "error code (0)"=w162) -> ("error out"=w153:errorcluster)  [unwired: 5 in]
        n53 = call <vilib>:"Add State(s) to Queue__JKI_lib_State_Machine.vi"("State(s) in (\"\")"=w158) -> ("States Out"=w157:string)  [unwired: 14 in]
      }
      frame "Initialize Core Data" {
        # "Do not delete, rename, or modify this frame.\n(this is used to determine panel behavior on exit)"
        # "originally closed?"
        # "exe?"
        # "If panel starts closed or is an EXE, then close it when we exit"
        n54 = property class="VI"() -> ("FP.State"=w166:T4)  [unwired: 2 in, 2 out]
        n55 = property class="App"() -> ("App.Kind"=w172:T5)  [unwired: 2 in, 2 out]
        n56 = control-ref of="Current VI Reference"() -> (w167:refnum<vi>)
        n57 = Equal?(x=w166, y=T4."Closed" ("Front Panel Window:State")) -> (x = y?=w164:bool)
        n58 = Equal?(x=w172, y=T5."Run Time System" ("Application:Kind")) -> (x = y?=w170:bool)
        n59 = Or(x=w164, y=w170) -> (x .or. y?=w168:bool)
        n60 = Bundle By Name(cluster=w169, "Core.Current VI Reference"=w167, "Core.Close Panel on Exit?"=w168) -> (w174:T8)
        n61 = call <vilib>:"Add State(s) to Queue__JKI_lib_State_Machine.vi"("State(s) in (\"\")"=w176) -> ("States Out"=w175:string)  [unwired: 14 in]
      }
      frame "Async Response", "Response" {
      }
      frame "Async Message Posted" {
      }
      frame "Exit" {
        # "Do not put any code in this frame.\n(No errors that occur here will be handled.)"
        n62 = call <vilib>:"Add State(s) to Queue__JKI_lib_State_Machine.vi"("State(s) in (\"\")"=w187) -> ("States Out"=w186:string)  [unwired: 14 in]
      }
      frame "---------- Data ----------" {
        # "Do not put any code in this frame.\n(It is a separator no-op. You can make a copy of this frame to create a new Data frame)"
        n63 = call <vilib>:"Add State(s) to Queue__JKI_lib_State_Machine.vi"("State(s) in (\"\")"=w191) -> ("States Out"=w190:string)  [unwired: 14 in]
      }
      frame "Data: Initialize" {
        w197 = u32 200  # SamplePeroid(ms)
        w198 = enum16{"Idle", "Acquiring"}."Idle"  # State
        w195 = T2 {"Resource"="", "SignalType"=enum."Sine Wave"}  # Configuration
        w199 = T7 {"Current VI Reference"=refnum, "Close Panel on Exit?"=FALSE}  # Core
        # "do not delete - used by framework"
        n64 = Bundle("Core"=w199, "Configuration"=w195, "State"=w198, "SamplePeroid(ms)"=w197) -> (w200:T8)  [unwired: 1 in]
        n65 = call "CSM - Read Cluster Elements From Session.vim"("Section Name (\"\" as Default)"=w196, "Cluster"=w195) -> ("error out"=w192:errorcluster, "Cluster out"=w193:T2)  [unwired: 6 in]
        n66 = Bundle By Name(cluster=w200, "Configuration"=w193) -> (w194:T8)
        n67 = call <vilib>:"Add State(s) to Queue__JKI_lib_State_Machine.vi"("State(s) in (\"\")"=w202) -> ("States Out"=w201:string)  [unwired: 14 in]
      }
      frame "Data: Update Indicators" {
        n68 = Unbundle By Name(w203) -> ("Configuration.SignalType"=w204:T3)
        n69 = local write "Signal Type"(w204) -> ()
      }
      frame "Data: Set Configuration" {
        n70 = call "Convert API String Arguments to Data.vim"("Reference Type"=w210, "API String"=w209) -> ("error out"=w207:errorcluster, "Data"=w208:T8)  [unwired: 6 in]
      }
      frame "Data: Get Configuration", "Data: Get Internal Data" {
        n71 = call "Query Data as API String Arguments.vim"("Name"=w214, "Cluster Data"=w216) -> ("error"=w212:errorcluster, "API String"=w213:string, "Cluster Data (dup)"=w215:T8)  [unwired: 7 in]
      }
      frame "Data: Cleanup" {
        # "Cleanup any data and references, here.\n(this is called automatically, by the Macro: Exit)"
        n72 = Unbundle By Name(w218) -> ("Core.Current VI Reference"=w221:refnum<vi>)
        n73 = Close Reference(reference=w221, error in (no error)=w220) -> (error out=w219:errorcluster)
        n74 = call <vilib>:"Add State(s) to Queue__JKI_lib_State_Machine.vi"("State(s) in (\"\")"=w223) -> ("States Out"=w222:string)  [unwired: 14 in]
      }
      frame "---------- Macro ----------" {
        # "Do not put any code in this frame.\n(It is a separator no-op. You can make a copy of this frame to create a new Macro frame)"
        n75 = call <vilib>:"Add State(s) to Queue__JKI_lib_State_Machine.vi"("State(s) in (\"\")"=w227) -> ("States Out"=w226:string)  [unwired: 14 in]
      }
      frame "Macro: Initialize" {
        # "Initialization Macro\n(This is called once, when the VI starts)"
        n76 = call <vilib>:"Add State(s) to Queue__JKI_lib_State_Machine.vi"("State(s) in Front (\"\")"="Data: Initialize\nInitialize Core Data\nData: Update Indicators", "State(s) in (\"\")"=w232) -> ("States Out"=w231:string)  [unwired: 13 in]
      }
      frame "Macro: Exit" {
        # "Exit Macro\n(This is called once, when the VI exits)"
        n77 = call <vilib>:"Add State(s) to Queue__JKI_lib_State_Machine.vi"("State(s) in Front (\"\")"="Data: Cleanup\nExit", "State(s) in (\"\")"=w237) -> ("States Out"=w236:string)  [unwired: 13 in]
      }
      frame "---------- API ----------" {
        # "Do not put any code in this frame.\n(It is a separator no-op. This category is recommended to use for external API)"
      }
      frame "API: Start" {
        # "#CSM-NOTE\nhttps://github.com/NEVSTOP-LAB/CSM-Continuous-Meausrement-and-Logging/issues/21\n\nUse CSM-Loop Support to define a loop in CSM, which is recommanded."
        # "Copy/Rename this case for your own API"
        n78 = Unbundle By Name(w246) -> ("State"=w247:enum16{"Idle", "Acquiring"})
        n79 = case shown="\"Idle\"" w247 {
          selector: w247 -> [w249 _]
          tunnel: [w249 enum16{"Idle", "Acquiring"}."Acquiring" ("Acquisition State")] -> w248
          tunnel: [_ "DAQ: Initialize \nDAQ: Configure\nDAQ: Start\nDAQ: Acquisite\nContinuous Check >> DAQ: Acquisite -><loop> \nDAQ: Stop\nDAQ: Close " ("State(s) in Front (\"\")")] -> w241
          frame "Acquiring" {
            # "The system is already acquiring. Ignore the \"Start\" message."
          }
          frame "Idle" {
            # "If the system is idle, start the acquisition."
          }
        }
        n80 = call <userlib>:"CSMLS - Define Loop State(s).vi"("Loop States"=w241, "States Queue"=w243) -> ("Remaining States"=w242:string)  [unwired: 13 in]
        n81 = Bundle By Name(cluster=w246, "State"=w248) -> (w245:T8)
      }
      frame "API: Stop" {
        # "Copy/Rename this case for your own API"
        n82 = Unbundle By Name(w252) -> ("State"=w257:enum16{"Idle", "Acquiring"})
        n83 = case shown="\"Acquiring\"" w257 {
          tunnel: ["Break Continuous" ("State(s) in Front (\"\")") _] -> w253
          frame "Acquiring" {
            # "If the system is acquiring, stop the acquisition."
          }
          frame "Idle" {
            # "The system is already idle. Ignore the \"Stop\" message."
          }
        }
        n84 = call <vilib>:"Add State(s) to Queue__JKI_lib_State_Machine.vi"("State(s) in Front (\"\")"=w253, "State(s) in (\"\")"=w256) -> ("States Out"=w255:string)  [unwired: 13 in]
      }
      frame "API: Update Settings" {
        # "#CSM-NOTE\nSync with ini-variable, to make sure the configuration could be stored in CSM INI-Variable configuration file."
        # "#CSM-NOTE\nUse this method to identify the argument type."
        n85 = Unbundle By Name(w267) -> ("Configuration"=w266:T2)
        n86 = call <userlib>:"CSM - Argument Type.vi"("Arguments"=w265) -> ("Argument Type"=w262:string, "Arguments (Dup)"=w263:string)  [unwired: 3 in]
        n87 = case shown="\"HexStr\"" w262 {
          tunnel: w266 -> [w272 w278]
          tunnel: [w271 w277] -> w259
          tunnel: [w270 w276] -> w264
          tunnel: w263 -> [w274 w275]
          frame "HexStr" {
            n88 = call <userlib>:"CSM - Convert HexStr to Data.vi"("HEX String"=w274) -> ("Variant"=w273:variant)  [unwired: 7 in, 1 out]
            n89 = Variant To Data(type=w272, Variant=w273) -> (data=w271:T2, error out=w270:errorcluster)  [unwired: 1 in]
          }
          frame Default {
            n90 = call "Convert API String Arguments to Data.vim"("Reference Type"=w278, "API String"=w275) -> ("error out"=w276:errorcluster, "Data"=w277:T2)  [unwired: 6 in]
          }
        }
        n91 = call "CSM - Write Configuration Variable.vim"("Section Name (\"\" as Default)"=w260, "error in (no error)"=w264, "Configuration"=w259) -> ("error out"=w261:errorcluster)  [unwired: 5 in, 1 out]
        n92 = Bundle By Name(cluster=w267, "Configuration"=w259) -> (w268:T8)
      }
      frame "---------- DAQ ----------" {
      }
      frame "DAQ: Initialize" {
        # "Edit these VIs to configure the acquisition."
        n93 = Unbundle By Name(w285) -> ("Configuration"=w286:T2)
        n94 = call "Initialize Hardware References.vi"("Hardware Resources in"=w286) -> ("error out"=w282:errorcluster, "Hardware Resources out"=w284:T2)  [unwired: 9 in]
        n95 = Bundle By Name(cluster=w285, "Configuration"=w284) -> (w283:T8)
      }
      frame "DAQ: Configure" {
        # "Edit these VIs to configure the acquisition."
        n96 = Unbundle By Name(w290) -> ("Configuration"=w292:T2)
        n97 = call "Configure Hardware.vi"("Hardware Resources in"=w292) -> ("error out"=w288:errorcluster, "Hardware Resources out"=w291:T2)  [unwired: 9 in]
        n98 = Bundle By Name(cluster=w290, "Configuration"=w291) -> (w289:T8)
      }
      frame "DAQ: Start" {
        w295 = u32 200  # SamplePeroid(ms)
        n99 = Bundle By Name(cluster=w297, "SamplePeroid(ms)"=w295, "State"=enum16{"Idle", "Acquiring"}."Acquiring" ("Acquisition State")) -> (w296:T8)
      }
      frame "DAQ: Acquisite" {
        n100 = Unbundle By Name(w305) -> ("State"=w309:enum16{"Idle", "Acquiring"})
        n101 = case shown="\"Acquiring\"" w309 {
          tunnel: [w311 w312] -> w307
          tunnel: w308 -> [w311 w316]
          tunnel: [w310 w317] -> w306
          tunnel: w305 -> [w310 w318]
          tunnel: [_ w314] -> w301
          frame "Idle" {
            # "Ignore \"Acquire\" messages when the acquisition is idle."
          }
          frame "Acquiring" {
            # "Edit these VIs to configure the acquisition."
            # "Acquire more data while in the \"Acquiring\" state."
            n102 = Unbundle By Name(w318) -> ("Configuration.Resource"=w319:string, "Configuration.SignalType"=w320:T3)
            n103 = call "Generate Simulated Data.vi"("error in (no error)"=w316, "Signal Type"=w320) -> ("error out"=w313:errorcluster, "Graph Data"=w315:waveform(dbl)[])  [unwired: 8 in]
            n104 = Bundle By Name(cluster=w318, "Configuration.Resource"=w319, "Configuration.SignalType"=w320) -> (w317:T8)
            n105 = call "CSM - Convert MassData to Argument.vim"("error in (no error)"=w313, "Data"=w315) -> ("error out"=w312:errorcluster, "MassData Argument"=w314:string)  [unwired: 6 in]
          }
        }
        n106 = call <vilib>:"Build State String with Arguments__JKI_lib_State_Machine.vi"("Arguments (\"\")"=w301, "State"="Acquired Waveform" ("Status with Arguments")) -> ("State with Arguments"=w300:string)  [unwired: 4 in]
        n107 = call <userlib>:"CSM - Broadcast Status Change.vi"("Status With Arguments"=w300, "State Queue"=w303) -> ("Remaining States"=w304:string)  [unwired: 13 in]
      }
      frame "DAQ: Stop" {
        n108 = Unbundle By Name(w323) -> ("Configuration"=w325:T2)
        n109 = call "Stop Acquisition.vi"("Hardware Resources in"=w325) -> ("error out"=w324:errorcluster)  [unwired: 10 in]
        n110 = Bundle By Name(cluster=w323, "State"=enum16{"Idle", "Acquiring"}."Idle" ("Acquisition State")) -> (w322:T8)
      }
      frame "DAQ: Close" {
      }
      frame "---------- Control Logic ----------" {
      }
      frame "Continuous Check" {
        n111 = Unbundle By Name(w336) -> ("SamplePeroid(ms)"=w335:u32)
        n112 = Wait (ms)(milliseconds to wait=w335) -> ()  [unwired: 1 out]
        n113 = call <userlib>:"CSMLS - Append Continuous State.vi"("Loop State(s) And Arguments"=w333, "Continous Arguments (\"\")"=w333, "Continous State"=w334, "States Queue"=w338) -> ("Remaining States"=w337:string)  [unwired: 7 in]
      }
      frame "Break Continuous" {
        n114 = call <userlib>:"CSMLS - Remove Loop Tag to Break.vi"("States Queue"=w341) -> ("Remaining States"=w340:string)  [unwired: 10 in]
      }
      frame "---------- DoSth ----------" {
      }
      frame "Do: Front Panel State" {
        n115 = Unbundle By Name(w351) -> ("Core.Current VI Reference"=w347:refnum<vi>)
        n116 = case shown="\"Hidden\", \"Hide\"" w349 {
          tunnel: w350 -> [w358 w373 w384 w397 w410]
          tunnel: [w360 w374 w386 w399 w412] -> w348
          tunnel: w347 -> [w359 w371 w385 w398 w411]
          frame "Open", "Standard", Default {
            w353 = T4."Standard" ("State")
            n117 = property class="VI"(reference=w359, error in=w358) -> (reference out=w356:refnum<vi>, error out=w357:errorcluster, "FP.State"=w355:T4)
            n118 = Not Equal?(x=w355, y=w353) -> (x != y?=w354:bool)
            n119 = case shown="True" w354 {
              tunnel: [w364 w366] -> w360
              tunnel: w357 -> [w363 w366]
              tunnel: w356 -> [w362 _]
              tunnel: w353 -> [w361 _]
              frame True {
                n120 = invoke class="VI" method="FP.Open"(reference=w362, error in=w363, "Activate"=TRUE, "State"=w361) -> (error out=w364:errorcluster)  [unwired: 1 in, 4 out]
              }
              frame False {
              }
            }
          }
          frame "Close", "Closed" {
            n121 = property class="VI"(reference=w371, error in=w373) -> (reference out=w370:refnum<vi>, error out=w372:errorcluster, "FP.State"=w368:T4)
            n122 = Not Equal?(x=w368, y=T4."Closed" ("Front Panel Window:State")) -> (x != y?=w367:bool)
            n123 = case shown="True" w367 {
              tunnel: [w375 w378] -> w374
              tunnel: w372 -> [w375 w377]
              tunnel: w370 -> [_ w376]
              frame False {
              }
              frame True {
                n124 = invoke class="VI" method="FP.Close"(reference=w376, error in=w377) -> (error out=w378:errorcluster)  [unwired: 1 in, 2 out]
              }
            }
          }
          frame "Hidden", "Hide" {
            w379 = T4."Hidden" ("State")
            n125 = property class="VI"(reference=w385, error in=w384) -> (reference out=w382:refnum<vi>, error out=w383:errorcluster, "FP.State"=w381:T4)
            n126 = Not Equal?(x=w381, y=w379) -> (x != y?=w380:bool)
            n127 = case shown="True" w380 {
              tunnel: [w390 w391] -> w386
              tunnel: w383 -> [w389 w391]
              tunnel: w382 -> [w388 _]
              tunnel: w379 -> [w387 _]
              frame True {
                n128 = invoke class="VI" method="FP.Open"(reference=w388, error in=w389, "State"=w387) -> (error out=w390:errorcluster)  [unwired: 2 in, 4 out]
              }
              frame False {
              }
            }
          }
          frame "Minimize", "Minimized" {
            w392 = T4."Minimized" ("State")
            n129 = property class="VI"(reference=w398, error in=w397) -> (reference out=w395:refnum<vi>, error out=w396:errorcluster, "FP.State"=w394:T4)
            n130 = Not Equal?(x=w394, y=w392) -> (x != y?=w393:bool)
            n131 = case shown="True" w393 {
              tunnel: [w403 w404] -> w399
              tunnel: w396 -> [w402 w404]
              tunnel: w395 -> [w401 _]
              tunnel: w392 -> [w400 _]
              frame True {
                n132 = invoke class="VI" method="FP.Open"(reference=w401, error in=w402, "State"=w400) -> (error out=w403:errorcluster)  [unwired: 2 in, 4 out]
              }
              frame False {
              }
            }
          }
          frame "Maximize", "Maximized" {
            w405 = T4."Maximized" ("State")
            n133 = property class="VI"(reference=w411, error in=w410) -> (reference out=w408:refnum<vi>, error out=w409:errorcluster, "FP.State"=w407:T4)
            n134 = Not Equal?(x=w407, y=w405) -> (x != y?=w406:bool)
            n135 = case shown="True" w406 {
              tunnel: [w416 w417] -> w412
              tunnel: w409 -> [w415 w417]
              tunnel: w408 -> [w414 _]
              tunnel: w405 -> [w413 _]
              frame True {
                n136 = invoke class="VI" method="FP.Open"(reference=w414, error in=w415, "State"=w413) -> (error out=w416:errorcluster)  [unwired: 2 in, 4 out]
              }
              frame False {
              }
            }
          }
        }
      }
      frame "Do: Hide FP and Exit When stand-alone" {
        # "#CSM-NOTE\nNo parent"
        n137 = Call Chain() -> (call chain=w424:string[])
        n138 = Array Size(array=w424) -> (size(s)=w423:i32)
        n139 = Equal?(x=1, y=w423) -> (x = y?=w421:bool)
        n140 = call-poly <userlib>:"Add State(s) to Queue By BOOL++.vi"("TRUE (\"\")"="Macro: Exit" ("State(s) at Back (\"\")"), "Condition"=w421, "State Queue (\"\")"="Do: Front Panel State >> Hide" ("State(s) at Back (\"\")")) -> ("Remaining States"=w418:string)  [unwired: 8 in]
        n141 = call <vilib>:"Add State(s) to Queue__JKI_lib_State_Machine.vi"("State(s) in Front (\"\")"=w418, "State(s) in (\"\")"=w419) -> ("States Out"=w420:string)  [unwired: 13 in]
      }
    }
  }
